vi "GetSystemChannelValues.vi"(8 "error in (no error)":errorcluster, 11 "VeriStandTestCase in":refnum<class "VeriStandTestCase.lvclass">) -> (0 "error out":errorcluster, 2 "System Channel Information":T1, 3 "VeriStandTestCase out":refnum<class "VeriStandTestCase.lvclass">)   [LabVIEW 2027, in "VeriStandTestCase.lvclass"]
uses:
  VeriStandTestCase.lvclass
  SystemChannelInformation.ctl
  VeriStandTestCase.lvclass/VeriStandTestCase.ctl
  <vilib>/NI VeriStand/Execution/Workspace/NI VeriStand - Get Multiple Channel Values.vi
  <vilib>/NI VeriStand/Execution/Workspace/NI_VS Workspace ExecutionAPI.lvlib
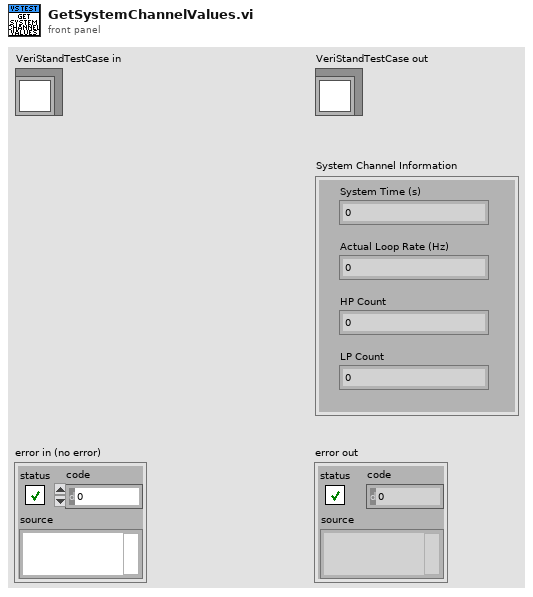
[diagram p1: front panel]
types:
  T1 = typedef "VeriStandTestCase.lvclass/SystemChannelInformation.ctl" = cluster{"Actual Loop Rate (Hz)":dbl, "System Time (s)":dbl, "HP Count":dbl, "LP Count":dbl}
  T2 = typedef "NI_VS Workspace ExecutionAPI.lvlib/WorkspaceAPI.ctl" = refnum<k39>
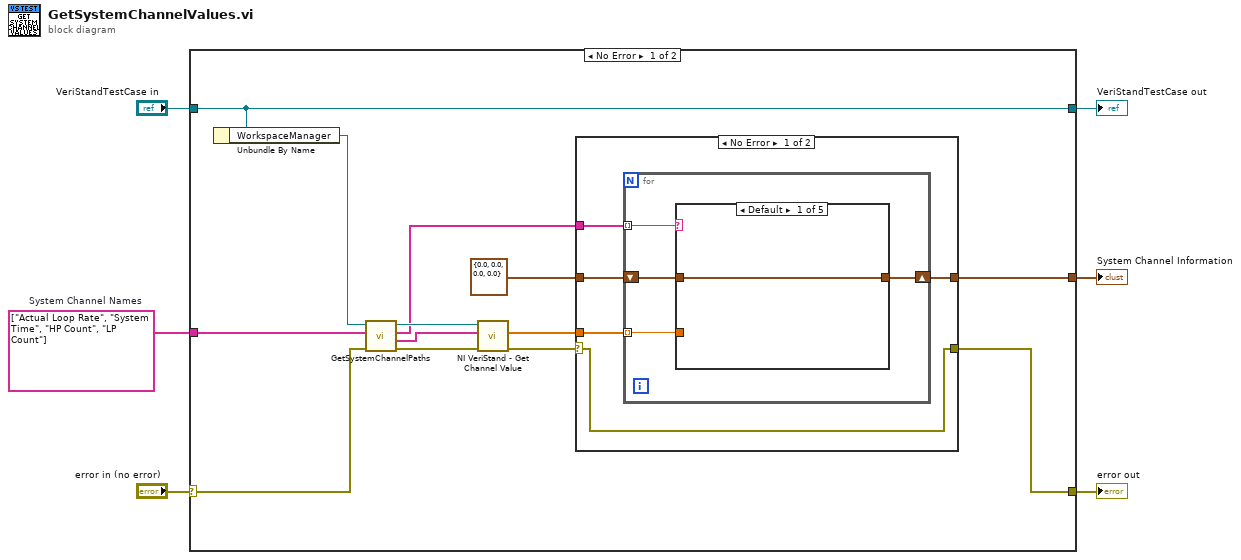
[diagram p0: block diagram]
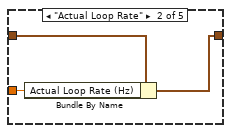
[diagram p2: hidden frame]
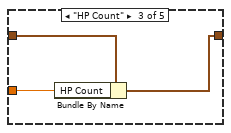
[diagram p3: hidden frame]
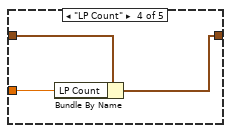
[diagram p4: hidden frame]
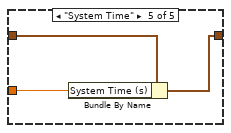
[diagram p5: hidden frame]
diagram:
  w2 = string[] ["Actual Loop Rate", "System Time", "HP Count", "LP Count"]  # System Channel Names
  n1 = case shown="No Error" "error in (no error)" {
    selector: "error in (no error)" -> [w18 w45]
    tunnel: [w10 w45] -> w5
    tunnel: [w19 w44] -> w3
    tunnel: "VeriStandTestCase in" -> [w19 w44]
    tunnel: w2 -> [w14 _]
    tunnel: [w11 _] -> w1
    frame No Error {
      n2 = Unbundle By Name(w19) -> ("WorkspaceManager"=w17:T2)
      n3 = call "GetSystemChannelPaths.vi"("error in (no error)"=w18, "System Channel Names in"=w14, "Workspace Manager Reference in"=w17) -> ("error out"=w16:errorcluster, "System Channel Full Paths out"=w13:string[], "System Channel Names out"=w12:string[], "Workspace Manager Reference out"=w15:T2)  [unwired: 5 in]
      n4 = call-poly <vilib>:"NI VeriStand - Get Channel Value.vi"("error in (no error)"=w16, "Channels"=w13, "WorkspaceManager in"=w15) -> ("error out"=w8:errorcluster, "Values"=w9:dbl[])  [unwired: 6 in, 1 out]
      n5 = case shown="No Error" w8 {
        selector: w8 -> [w20 w42]
        tunnel: w9 -> [w24 _]
        tunnel: w12 -> [w23 _]
        tunnel: [w22 w43] -> w11
        tunnel: T1 {"Actual Loop Rate (Hz)"=0.0, "System Time (s)"=0.0, "HP Count"=0.0, "LP Count"=0.0} ("System Channel Information") -> [w21 w43]
        tunnel: [w20 w42] -> w10
        frame No Error {
          n6 = for {
            tunnel: w24 -> [w27] mode=indexing
            tunnel: w23 -> [w28] mode=indexing
            shift-right: [w26] -> w22
            shift-left: w21 -> [w25]
            n7 = case shown="Default" w28 {
              tunnel: w27 -> [_ w30 w33 w36 w39]
              tunnel: [w29 w31 w34 w37 w40] -> w26
              tunnel: w25 -> [w29 w32 w35 w38 w41]
              frame Default {
              }
              frame "Actual Loop Rate" {
                n8 = Bundle By Name(cluster=w32, "Actual Loop Rate (Hz)"=w30) -> (w31:T1)
              }
              frame "HP Count" {
                n9 = Bundle By Name(cluster=w35, "HP Count"=w33) -> (w34:T1)
              }
              frame "LP Count" {
                n10 = Bundle By Name(cluster=w38, "LP Count"=w36) -> (w37:T1)
              }
              frame "System Time" {
                n11 = Bundle By Name(cluster=w41, "System Time (s)"=w39) -> (w40:T1)
              }
            }
          }
        }
        frame Error {
        }
      }
    }
    frame Error {
    }
  }
  "error out" <- w5
  "VeriStandTestCase out" <- w3
  "System Channel Information" <- w1
